vi "pb-start.vi"(11 "path in":path=path "C:/SpinCore/SpinAPI/dll/spinapi64.dll") -> (3 "path out":path)   [LabVIEW 2018]
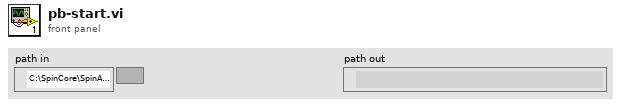
[diagram p1: front panel]
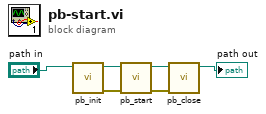
[diagram p0: block diagram]
diagram:
  n1 = call "pb_init.vi"("path in"="path in") -> ("error out"=w3:errorcluster, "path out"=w4:path)  [unwired: 9 in]
  n2 = call "pb_start.vi"("error in (no error)"=w3, "path in"=w4) -> ("error out"=w5:errorcluster, "path out"=w6:path)  [unwired: 8 in]
  n3 = call "pb_close.vi"("error in (no error)"=w5, "path in"=w6) -> ("path out"=→"path out":path)  [unwired: 8 in, 1 out]
